vi "Find and Init ESP300.vi"(8 "error in (no error)":errorcluster, 10 "A Valid Axis":i32=1) -> (0 "error out":errorcluster, 3 "VISA resource name out":refnum<visa-resource-name>)   [LabVIEW 2015]
uses:
  <vilib>/Instr/_visa.llb/VISA Find Search Mode.ctl
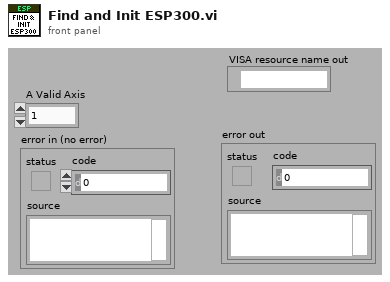
[diagram p1: front panel]
types:
  T1 = typedef "VISA Find Search Mode.ctl" = u32
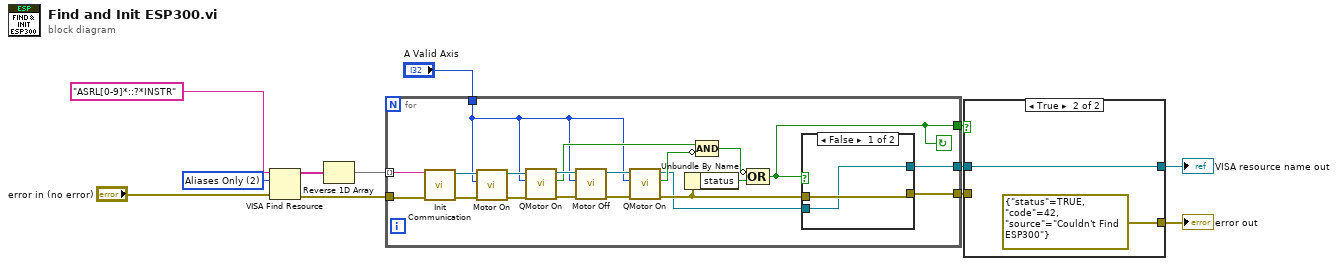
[diagram p0: block diagram]
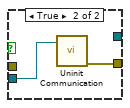
[diagram p3: hidden frame]
diagram:
  w12 = T1 2 items=["Canonical Names Only"=0, "Aliases Only"=2, "Include Matching Aliases"=3, "Include All Aliases"=4] ("Search Mode")
  n1 = VISA Find Resource(8:"error in (no error)", 10:w12, 11:"ASRL[0-9]*::?*INSTR" ("expression (\"?*\")")) -> (0:w9:errorcluster, 3:w10:string[])  [unwired: 1 out]
  n2 = Reverse 1D Array(array=w10) -> (reversed array=w2:string[])
  n3 = for {
    tunnel: w2 -> [w32] mode=indexing
    tunnel: w9 -> [w31]
    tunnel: [w17] -> w8
    tunnel: [w15] -> w7
    tunnel: [w14] -> w6
    tunnel: "A Valid Axis" -> [w13]
    stop <- w17 continue-if-true
    n4 = call "Init Communication.vi"("error in (no error)"=w31, "VISA resource name in"=w32) -> ("error out"=w29:errorcluster, "VISA resource name out"=w30:refnum<visa-resource-name>)  [unwired: 8 in]
    n5 = call "Motor On.vi"("error in (no error)"=w29, "Axis"=w13, "VISA resource name in"=w30) -> ("error out"=w27:errorcluster, "VISA resource name out"=w28:refnum<visa-resource-name>)  [unwired: 7 in]
    n6 = call "QMotor On.vi"("error in (no error)"=w27, "Axis"=w13, "VISA resource name in"=w28) -> ("error out"=w25:errorcluster, "Motor On?"=w22:bool, "VISA resource name out"=w26:refnum<visa-resource-name>)  [unwired: 6 in]
    n7 = call "Motor Off.vi"("error in (no error)"=w25, "Axis"=w13, "VISA resource name in"=w26) -> ("error out"=w23:errorcluster, "VISA resource name out"=w24:refnum<visa-resource-name>)  [unwired: 7 in]
    n8 = call "QMotor On.vi"("error in (no error)"=w23, "Axis"=w13, "VISA resource name in"=w24) -> ("error out"=w18:errorcluster, "Motor On?"=w21:bool, "VISA resource name out"=w16:refnum<visa-resource-name>)  [unwired: 6 in]
    n9 = Unbundle By Name(w18) -> ("status"=w20:bool)
    n10 = Compound Arithmetic op=AND(w22, invert w21) -> (w19:bool)
    n11 = Compound Arithmetic op=OR(invert w19, w20) -> (w17:bool)
    n12 = case shown="False" w17 {
      tunnel: w18 -> [w34 _]
      tunnel: w16 -> [w33 w36]
      tunnel: [w34 w35] -> w15
      tunnel: [w33 _] -> w14
      frame False {
      }
      frame True {
        n13 = call "Uninit Communication.vi"("VISA resource name in"=w36) -> ("error out"=w35:errorcluster)  [unwired: 10 in]
      }
    }
  }
  n14 = case shown="True" w8 {
    tunnel: w7 -> [w38 _]
    tunnel: w6 -> [w37 w40]
    tunnel: [w37 w40] -> w5
    tunnel: [w38 errorcluster {"status"=TRUE, "code"=42, "source"="Couldn't Find ESP300"} ("error out")] -> w4
    frame False {
    }
    frame True {
    }
  }
  "VISA resource name out" <- w5
  "error out" <- w4
